vi "SubVI_CreateNewVI.vi"(8 "error in (no error)":errorcluster, 11 "vi path":string) -> (0 "error out":errorcluster, 3 "VI out":refnum<vi>)   [LabVIEW 2015]
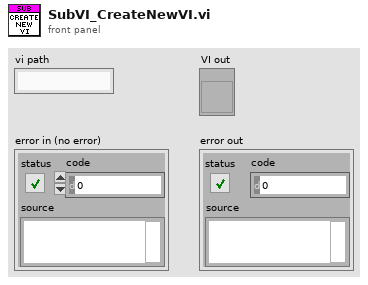
[diagram p1: front panel]
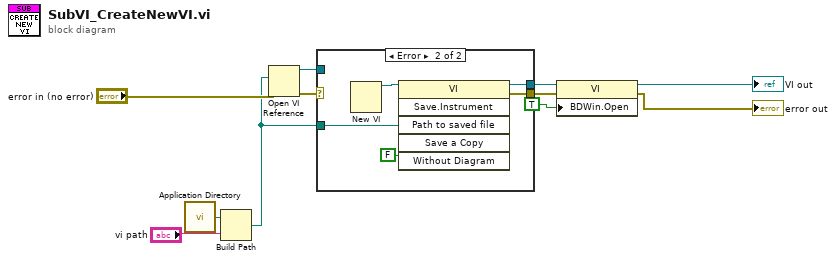
[diagram p0: block diagram]
diagram:
  n1 = call <vilib>:"Application Directory.vi"() -> ("Application Directory"=w3:path)
  n2 = Build Path(base path=w3, name or relative path="vi path") -> (appended path=w5:path)
  n3 = Open VI Reference(vi path=w5, error in (no error)="error in (no error)") -> (vi reference=w8:refnum<vi>, error out=w9:errorcluster)  [unwired: 4 in]
  n4 = case shown="Error" w9 {
    selector: w9 -> [w12 _]
    tunnel: w5 -> [_ w16]
    tunnel: [w13 w14] -> w6
    tunnel: w8 -> [w13 _]
    tunnel: [w12 w15] -> w7
    frame No Error {
    }
    frame Error {
      n5 = New VI() -> (3:w18:refnum<vi>)  [unwired: 7 in, 1 out]
      n6 = invoke class="VI" method="Save.Instrument"(reference=w18, "Path to saved file"=w16, "Without Diagram"=FALSE) -> (reference out=w14:refnum<vi>, error out=w15:errorcluster)  [unwired: 3 in, 4 out]
    }
  }
  n7 = property class="VI"(reference=w6, error in=w7, "BDWin.Open"=TRUE ("Block Diagram Window:Open")) -> (reference out=→"VI out":refnum<vi>, error out=→"error out":errorcluster)
